vi "HT3_ByteArrayToStrs.vi"(10 "Byte Array":u8[](array[numeric]), 11 "Lengths":i32[](array[numeric])) -> (2 "Strings":string[](array[string]))   [LabVIEW 2010]
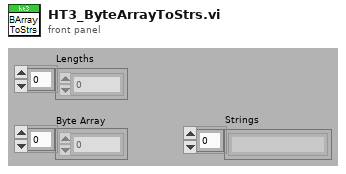
[diagram p1: front panel]
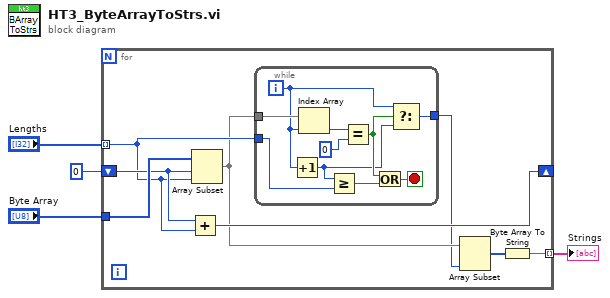
[diagram p0: block diagram]
diagram:
  n1 = for {
    tunnel: "Lengths" -> [w9] mode=indexing
    tunnel: "Byte Array" -> [w12]
    shift-right: [w10] -> _
    shift-left: 0 ("index") -> [w11]
    tunnel: [w5] -> w1 mode=indexing
    n2 = Add(x=w11, y=w9) -> (x+y=w10:i32)
    n3 = Array Subset(array=w12, index=w11, length=w9) -> (w8:u8[])
    n4 = while {
      tunnel: w8 -> [w22]
      tunnel: w9 -> [w17]
      tunnel: [w13] -> w7
      i -> [w15]
      stop <- w19 stop-if-true
      n5 = Increment(x=w15) -> (x+1=w14:i32)
      n6 = Index Array(array=w22, index=w15) -> (element=w21:u8)
      n7 = Greater Or Equal?(x=w14, y=w17) -> (x >= y?=w18:bool)
      n8 = Equal?(x=w21, y=u8 0) -> (x = y?=w16:bool)
      n9 = Or(x=w16, y=w18) -> (x .or. y?=w19:bool)
      n10 = Select(t=w15, s=w16, f=w14) -> (s? t:f=w13:i32)
    }
    n11 = Array Subset(array=w8, length=w7) -> (w6:u8[])  [unwired: 1 in]
    n12 = Byte Array To String(unsigned byte array=w6) -> (string=w5:string)
  }
  "Strings" <- w1
